vi "HighSpeedAveragevi.vi"(8 "input valid":bool=TRUE, 10 "y":fxp<+/-,16,14>, 11 "x":fxp<+/-,16,14>) -> (0 "output valid":bool, 3 "(x+y)/2":fxp<+/-,16,14>)   [LabVIEW 2018]
uses:
  <vilib>/rvi/FXPMathLib/FxpConvert/subVIs/nifxpmath_Convert_SimConfig.ctl
  <vilib>/fxp/LVFixedPointQuantizationPolicyTypeDef.ctl
  <vilib>/fxp/LVFixedPointOverflowPolicyTypeDef.ctl
  <vilib>/rvi/FXPMathLib/FxpConvert/simVIs/DllFxpConvertTemp_sub.vi
  <vilib>/rvi/FXPMathLib/FxpConvert/XNode/nifxpmath_Convert.xnode
  <vilib>/rvi/FXPMathLib/FxpInterpret/XNode/nifxpmath_Interpret.xnode
  <vilib>/rvi/FXPMathLib/FxpAdd/XNode/nifxpmath_Add.xnode
  <vilib>/rvi/FXPMathLib/sim/FxpSim.dll
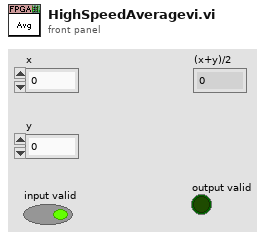
[diagram p1: front panel]
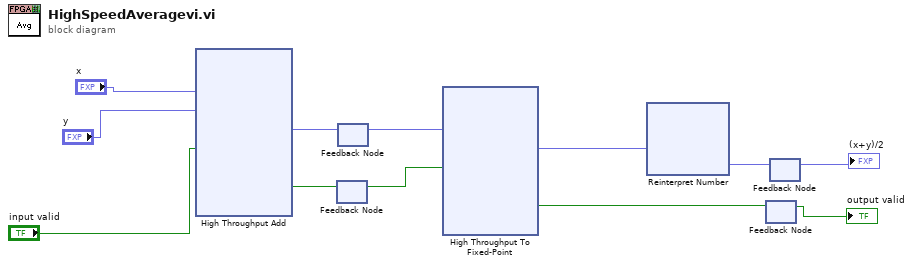
[diagram p0: block diagram]
diagram:
  n1 = xnode ("High Throughput Add")("x"="x", "y"="y", "input valid"="input valid") -> ("x+y"=w12:fxp<+/-,17,15>, "output valid"=w11:bool)  [unwired: 1 in, 1 out]
  n2 = feedback #1() -> (w6:bool)  [unwired: 1 in]
  n3 = feedback-in #1(w11) -> ()
  n4 = feedback #2() -> (w7:fxp<+/-,17,15>)  [unwired: 1 in]
  n5 = feedback-in #2(w12) -> ()
  n6 = xnode "High Throughput To Fixed-Point"("x"=w7, "input valid"=w6) -> ("y"=w5:fxp<+/-,16,15>, "output valid"=w3:bool)  [unwired: 1 in, 1 out]
  n7 = xnode "Reinterpret Number"("x"=w5) -> ("y"=w4:fxp<+/-,16,14>)
  n8 = feedback #3() -> (→"output valid":bool)  [unwired: 1 in]
  n9 = feedback-in #3(w3) -> ()
  n10 = feedback #4() -> (→"(x+y)/2":fxp<+/-,16,14>)  [unwired: 1 in]
  n11 = feedback-in #4(w4) -> ()
